vi "ConfigUtilities - Get Items Names.vi"(8 "error IO 2":errorcluster, 11 "TCP Channel Refs In":T1[](array[typedef]) format="%.0x") -> (0 "error IO":errorcluster, 1 "Items Names":string[][](array[string]), 3 "TCP Channel Refs Out":T1[](array[typedef]) format="%.0x")   [LabVIEW 2016, in "UDP-Custom-Device System Explorer.lvlib"]
doc: "Gets multiple channel names and paths."
uses:
  UDP-Custom-Device System Explorer.lvlib
  <vilib>/NI Veristand/Custom Device API/Custom Device Item Ref.ctl
  <vilib>/NI VeriStand/Custom Device API/Custom Device API.lvlib
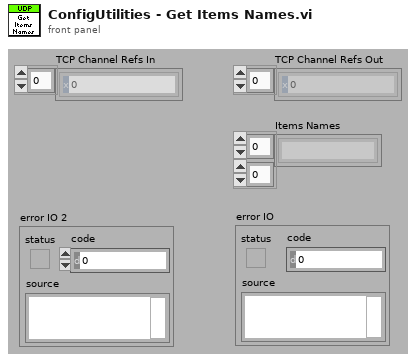
[diagram p1: front panel]
types:
  T1 = typedef "Custom Device API.lvlib/Custom Device Item Ref.ctl" = u64
  T2 = typedef "Custom Device API.lvlib/Custom Device Item Info.ctl" = cluster{"Name":string, "Is Channel":bool, "GUID":string, "Is Waveform":bool}
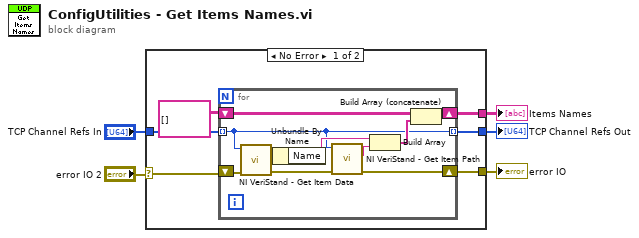
[diagram p0: block diagram]
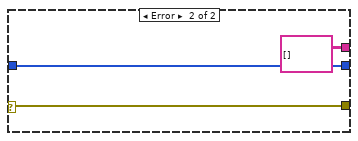
[diagram p2: hidden frame]
diagram:
  n1 = case shown="No Error" "error IO 2" {
    selector: "error IO 2" -> [w6 w23]
    tunnel: [w11 w23] -> w5
    tunnel: [w10 string[][] []] -> w4
    tunnel: [w8 w24] -> w3
    tunnel: "TCP Channel Refs In" -> [w7 w24]
    frame No Error {
      n2 = for {
        tunnel: w7 -> [w12] mode=indexing
        tunnel: [w12] -> w8 mode=indexing
        shift-right: [w19] -> w11
        shift-left: w6 -> [w21]
        shift-right: [w14] -> w10
        shift-left: string[][] [] -> [w13]
        n3 = call <vilib>:"NI VeriStand - Get Item Data.vi"("error in (no error)"=w21, "Item Ref in"=w12) -> ("error out"=w20:errorcluster, "Item Info"=w18:T2)  [unwired: 6 in, 2 out]
        n4 = Unbundle By Name(w18) -> ("Name"=w16:string)
        n5 = call <vilib>:"NI VeriStand - Get Item Path.vi"("error in (no error)"=w20, "Item Ref in"=w12) -> ("error out"=w19:errorcluster, "Path"=w17:string)  [unwired: 8 out]
        n6 = Build Array(w16, w17) -> (w15:string[])
        n7 = Build Array (concatenate)(w13, w15) -> (w14:string[][])
      }
    }
    frame Error {
    }
  }
  "error IO" <- w5
  "Items Names" <- w4
  "TCP Channel Refs Out" <- w3
